vi "LVClass_ComputePhaseSet equalize AB.vi"(0 "ComputePhaseSet dest in":refnum<class "ComputePhaseSet.lvclass">, 5 "ComputePhaseSet source in":refnum<class "ComputePhaseSet.lvclass">, 11 "error in (no error)":errorcluster) -> (4 "ComputePhaseSet dest out":refnum<class "ComputePhaseSet.lvclass">, 15 "error out":errorcluster)   [LabVIEW 2020, in "ComputePhaseSet.lvclass"]
doc: "Deep copy.\n\n<B>ComputePhaseSet_dstIn</B> : ComputePhaseSet object to assign.\n<B>ComputePhaseSet_dstOut</B> : ComputePhaseSet object to assign.\n<B>ComputePhaseSet_src</B> : ComputePhaseSet object to copy."
uses:
  ComputePhaseSet.lvclass
  WavefrontReconstructionMode.ctl
  Handle creation.ctl
  ComputePhaseSet.lvclass/ComputePhaseSet.ctl
  LVClass_ComputePhaseSet Read ComputePhaseSet.vi
panel:
  out "Reconstruction Mode":T1=enum."Modal_Legendre"
  out "ComputePhaseSet source out":refnum<class "ComputePhaseSet.lvclass">
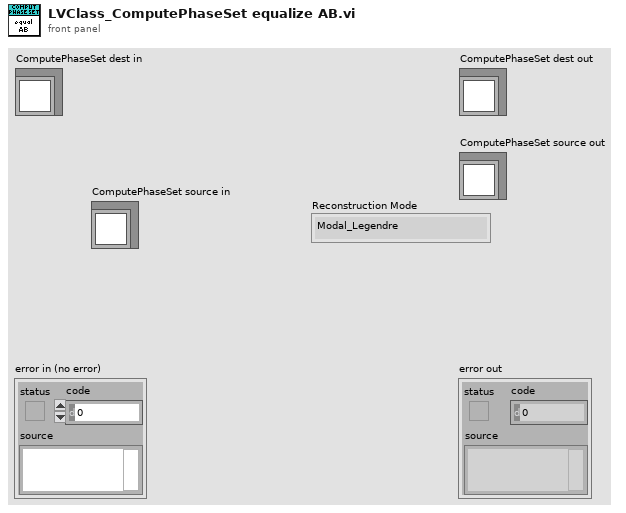
[diagram p1: front panel]
types:
  T1 = typedef "WavefrontReconstructionMode.ctl" = enum16{"None", "Modal_Legendre", "Modal_Zernike", "Zonal", "Modal_Zonal_Zernike", "Modal_Zonal_Legendre"}
  T2 = typedef "Handle creation.ctl" = enum16{"By ctor", "By write function"}
  T3 = typedef "ClassID.ctl" = i64
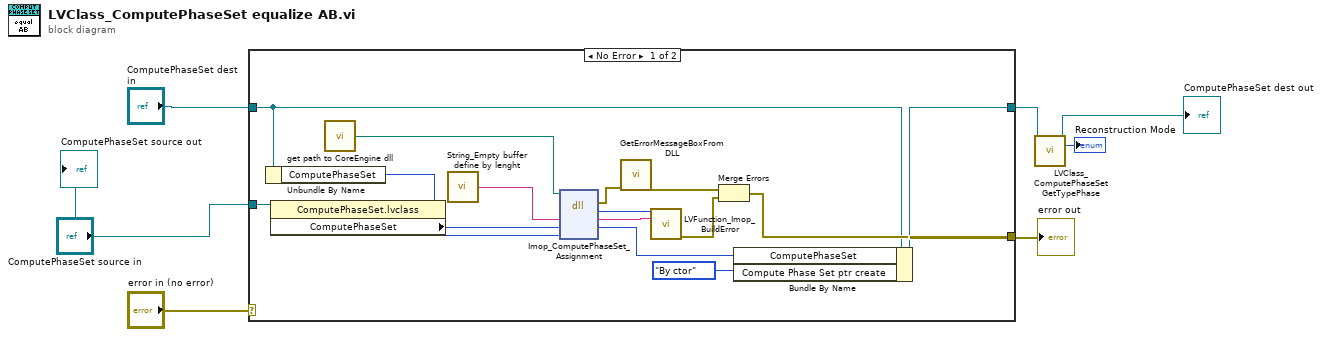
[diagram p0: block diagram]
diagram:
  n1 = case shown="No Error" "error in (no error)" {
    selector: "error in (no error)" -> [_ w24]
    tunnel: [w12 w24] -> w5
    tunnel: [w18 w23] -> w3
    tunnel: "ComputePhaseSet dest in" -> [w9 w23]
    tunnel: "ComputePhaseSet source in" -> [w11 _]
    frame No Error {
      n2 = Unbundle By Name(w9) -> ("ComputePhaseSet"=w8:T3)
      n3 = property class="ComputePhaseSet.lvclass"(reference=w11) -> ("ComputePhaseSet"=w10:T3)  [unwired: 1 in, 2 out]
      n4 = call "get path to CoreEngine dll.vi"() -> ("path to wavekit library"=w16:path)  [unwired: 14 in, 1 out]
      n5 = call "String_Empty buffer define by lenght.vi"() -> ("Empty buffer"=w17:string)  [unwired: 1 in]
      n6 = dll-call lib="D:/soft/HASO_v3/SVN_trunk/ImOpCoreEngine4_LV2011/DLLs/c_interface_vc100.dll" fn="Imop_ComputePhaseSet_Assignment"(path in=w16, "message"=w17, "ComputePhaseSet Dest"=w8, "ComputePhaseSet Source"=w10) -> (error out=w15:errorcluster, "return type"=w21:i32, "message"=w20:string, "ComputePhaseSet Dest"=w19:i64)  [unwired: 3 in, 1 out]
      n7 = call "GetErrorMessageBoxFromDLL.vi"("error IN"=w15) -> ("error OUT"=w14:errorcluster)  [unwired: 10 in]
      n8 = call "LVFunction_Imop_BuildError.vi"("code"=w21, "String to Prepend to source (\"\")"=w20) -> ("error out"=w13:errorcluster)  [unwired: 13 in]
      n9 = Merge Errors(w14, w13) -> (w12:errorcluster)
      n10 = Bundle By Name(cluster=w9, "ComputePhaseSet"=w19, "Compute Phase Set ptr create"=Handle_creation."By ctor" ("Haso ptr create")) -> (w18:refnum<class "ComputePhaseSet.lvclass">)
    }
    frame Error {
    }
  }
  "error out" <- w5
  n11 = call "LVClass_ComputePhaseSet GetTypePhase.vi"("ComputePhaseSet in"=w3) -> ("ComputePhaseSet out"=→"ComputePhaseSet dest out":refnum<class "ComputePhaseSet.lvclass">, "Reconstruction Mode"=→"Reconstruction Mode":T1)  [unwired: 12 in, 1 out]
  "ComputePhaseSet source out" <- "ComputePhaseSet source in"
